vi "Modify Index based on Datavalid (4 inputs).vi"(7 "previous counter val":T1, 9 "cuurent index data valid?":bool, 10 "Actual Index":T1) -> (1 "Next Counter Val":T1, 2 "Modified Index":T1)   [LabVIEW 2011]
uses:
  <userlib>/FPGA Library/Code Development/Signal Processing/Input Multiplexer to FFT/4 Input MUX/Input Index(Type) 4 inputs.ctl
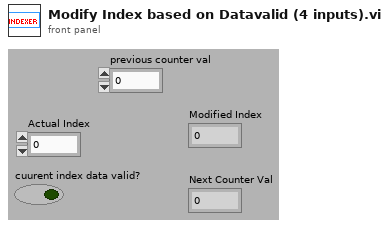
[diagram p1: front panel]
types:
  T1 = typedef "Input Index(Type) 4 inputs.ctl" = fxp<+,2,2>
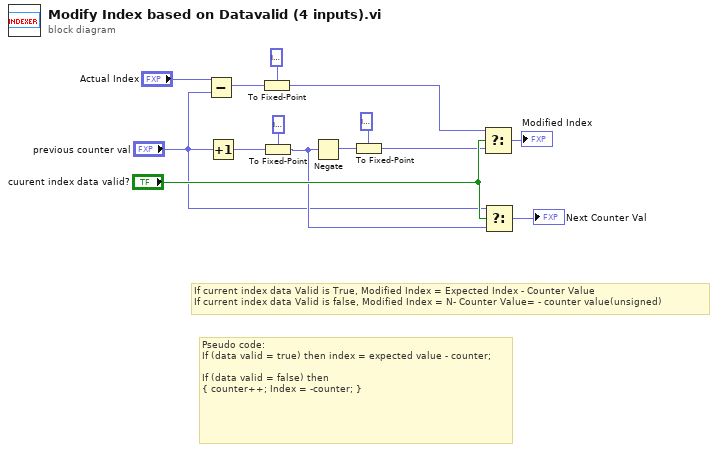
[diagram p0: block diagram]
diagram:
  # "Pseudo code:\nIf (data valid = true) then index = expected value - counter;\n\nIf (data valid = false) then \n{ counter++; Index = -counter; }"
  # "If current index data Valid is True, Modified Index = Expected Index - Counter Value                         \nIf current index data Valid is false, Modified Index = N- Counter Value= - counter value(unsigned)"
  n1 = Subtract(x="Actual Index", y="previous counter val") -> (x-y=w10:fxp<+/-,3,3>)
  n2 = Increment(x="previous counter val") -> (x+1=w7:fxp<+,3,3>)
  n3 = To Fixed-Point(fixed-point type=T1 0.0 ("Actual Index"), number=w10) -> (fixed-point=w8:T1)
  n4 = To Fixed-Point(fixed-point type=T1 0.0 ("Actual Index"), number=w7) -> (fixed-point=w2:T1)
  n5 = Negate(x=w2) -> (-x=w5:fxp<+/-,3,3>)
  n6 = To Fixed-Point(fixed-point type=T1 0.0 ("Actual Index"), number=w5) -> (fixed-point=w3:T1)
  n7 = Select(t=w8, s="cuurent index data valid?", f=w3) -> (s? t:f=→"Modified Index":T1)
  n8 = Select(t="previous counter val", s="cuurent index data valid?", f=w2) -> (s? t:f=→"Next Counter Val":T1)
